vi "Configure Power Analysis (Transient).vi"(7 "New Load Current Value (0.215 A)":dbl=0.215, 8 "error in (no error)":errorcluster, 9 "Initial Current Value (0.06 A)":dbl=0.06, 10 "Operation (0: Apply)":i32(ring) items=["Apply", "Exit", "Go to Next Step", "Specify Initial Load Current Value", "Specify New Load Current Value"], 11 "VISA resource name":refnum<visa-resource-name>) -> (0 "error out":errorcluster, 3 "VISA resource name out":refnum<visa-resource-name>)   [LabVIEW 2023, in "Keysight-DSQx3014T.lvlib"]
doc: "Applies the transient analysis."
uses:
  Keysight-DSQx3014T.lvlib
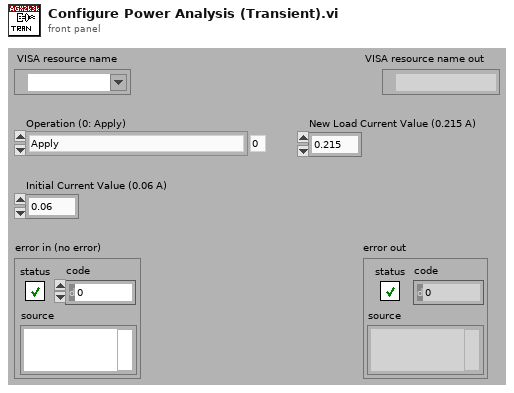
[diagram p1: front panel]
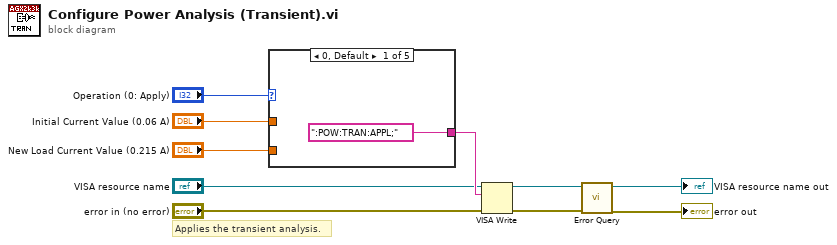
[diagram p0: block diagram]
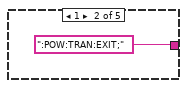
[diagram p2: hidden frame]
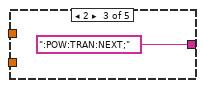
[diagram p3: hidden frame]
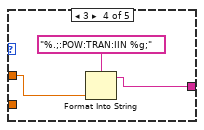
[diagram p4: hidden frame]
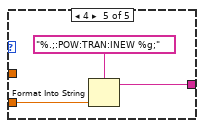
[diagram p5: hidden frame]
diagram:
  # "Applies the transient analysis."
  n1 = case shown="0, Default" "Operation (0: Apply)" {
    tunnel: [":POW:TRAN:APPL;" ":POW:TRAN:EXIT;" ":POW:TRAN:NEXT;" w14 w18] -> w5
    tunnel: "Initial Current Value (0.06 A)" -> [_ _ _ w16 _]
    tunnel: "New Load Current Value (0.215 A)" -> [_ _ _ _ w17]
    frame 0, Default {
    }
    frame 1 {
    }
    frame 2 {
    }
    frame 3 {
      n2 = Format Into String(format string="%.;:POW:TRAN:IIN %g;", w16) -> (resulting string=w14:string)  [unwired: 2 in, 1 out]
    }
    frame 4 {
      n3 = Format Into String(format string="%.;:POW:TRAN:INEW %g;", w17) -> (resulting string=w18:string)  [unwired: 2 in, 1 out]
    }
  }
  n4 = VISA Write(VISA resource name="VISA resource name", write buffer=w5, error in (no error)="error in (no error)") -> (VISA resource name out=w10:refnum<visa-resource-name>, error out=w9:errorcluster)  [unwired: 1 out]
  n5 = call "Error Query.vi"("error in (no error)"=w9, "VISA resource name"=w10) -> ("error out"=→"error out":errorcluster, "VISA resource name out"=→"VISA resource name out":refnum<visa-resource-name>)  [unwired: 8 out]
